vi "DemoVI_Thingworx.vi"() -> ()   [LabVIEW 2018]
panel:
  out "Thingworx Timestamp String":string="1557144000000"
  out "ThingworxTimestamp":dbl=1557144000000.0 format="%#_19g"
  out "Unix Timestamp":dbl=1557144000.0 format="%#_16g"
  in  "Labview Timestamp":timestamp=timestamp(3639960000 s since 1904-01-01) format="%<%H:%M:%S%3u\n%x>T"
  in  "Outer JSON":string
  in  "Inner JSON":string="StringField"
  in  "Outer JSON":string="rows"
  out "Complete Request URL":string="http://192.168.1.144:80/Thingworx/Things/LabviewTestObject/Properties/StringField"
  out "REST Answer as JSON 4":string="{\"dataShape\":{\"fieldDefinitions\":{\"result\":{\"name\":\"result\",\"description\":\"\",\"baseType\":\"STRING\",\"ordinal\":0,\"aspects\":{}}}},\"rows\":[{\"result\":\"input correct - service executed\"}]}"
  out "error out":errorcluster={"status"=FALSE, "code"=200, "source"="HTTP OK"}
  out "parsed JSON result --- jsonObject.row[0].result":string="input correct - service executed"
  in  "Thingworx Server Information":T1={"Server Adress"="192.168.1.144", "Port"="80", "http / https"="http", "Application Key"="8f240f9e-5025-45fe-9253-3b420d7beb56", "Entity Collection"="Things", "Name of Entity"="LabviewTestObject", "Characteristic Collection"="Services", "Name of Characteristic"="TestService", "Request Method"=enum."POST", "JSON Request Body"="{\n\"contentCheck\" : true\n}"}
  out "REST Answer as JSON 3":string="{\"dataShape\":{\"fieldDefinitions\":{\"result\":{\"name\":\"result\",\"description\":\"result\",\"baseType\":\"STRING\",\"ordinal\":0,\"aspects\":{}}}},\"rows\":[{\"result\":\"RUNNING\"}]}"
  out "error out":errorcluster={"status"=FALSE, "code"=200, "source"="HTTP OK"}
  out "parsed JSON result --- jsonObject.row[0].result":string="RUNNING"
  in  "Thingworx Server Information":T1={"Server Adress"="192.168.1.144", "Port"="80", "http / https"="http", "Application Key"="8f240f9e-5025-45fe-9253-3b420d7beb56", "Entity Collection"="Subsystems", "Name of Entity"="PlatformSubsystem", "Characteristic Collection"="Services", "Name of Characteristic"="GetSubsystemState", "Request Method"=enum."POST", "JSON Request Body"=""}
  out "REST Answer as JSON 2":string="{}"
  out "error out":errorcluster
  out "parsed JSON result --- not possible for put":string="***no result***"
  in  "Thingworx Server Information":T1={"Server Adress"="192.168.1.144", "Port"="80", "http / https"="http", "Application Key"="8f240f9e-5025-45fe-9253-3b420d7beb56", "Entity Collection"="Things", "Name of Entity"="LabviewTestObject", "Characteristic Collection"="Properties", "Name of Characteristic"="Timestamp", "Request Method"=enum."PUT", "JSON Request Body"="************This will be overwritten with the created Timestamp*********"}
  out "REST Answer as JSON":string="{\"dataShape\":{\"fieldDefinitions\":{\"StringField\":{\"name\":\"StringField\",\"description\":\"\",\"baseType\":\"STRING\",\"ordinal\":3,\"aspects\":{\"isPersistent\":true,\"dataChangeType\":\"VALUE\",\"cacheTime\":0.0}}}},\"rows\":[{\"StringField\":\"Custom String\"}]}"
  out "error out":errorcluster={"status"=FALSE, "code"=200, "source"="HTTP OK"}
  out "parsed JSON result --- jsonObject.rows[0].StringField":string="Custom String"
  in  "Thingworx Server Information":T1={"Server Adress"="192.168.1.144", "Port"="80", "http / https"="http", "Application Key"="8f240f9e-5025-45fe-9253-3b420d7beb56", "Entity Collection"="Things", "Name of Entity"="LabviewTestObject", "Characteristic Collection"="Properties", "Name of Characteristic"="StringField", "Request Method"=enum."GET", "JSON Request Body"=""}
  # "Demonstration of a GET call to retrieve propery values from Thingworx"
  # "Demonstration of a PUT call to set propery values in Thingworx"
  # "Demonstration of a POST call to execute a Thingworx service"
  # "Demonstration of a POST call to execute a Thingworx service with request body"
  # "If Outer JSON is empty, no JSON evaluation happens"
  # "The Thingworx Timestamp is the UNIX timestamp * 1000 to have the timestamp\nin milliseconds.\nThe epoch of Thingworx is 1/1/1970 in MS; the epoch of LabVIEW is 1/1/1904.\nTo help convert the dates, the SubVI Helper_Timestamp will do the transformation."
  # "Inner JSON and Outer JSON can be used to navigate \ndifferent than rows[0].result"
  # "Thingworx REST - Learning Guide"
  # "https://developer.thingworx.com/en/resources/guides/thingworx-rest-api-quickstart"
  # "Thingworx REST API Pattern"
  # "Thingworx REST API HTTP request verbs"
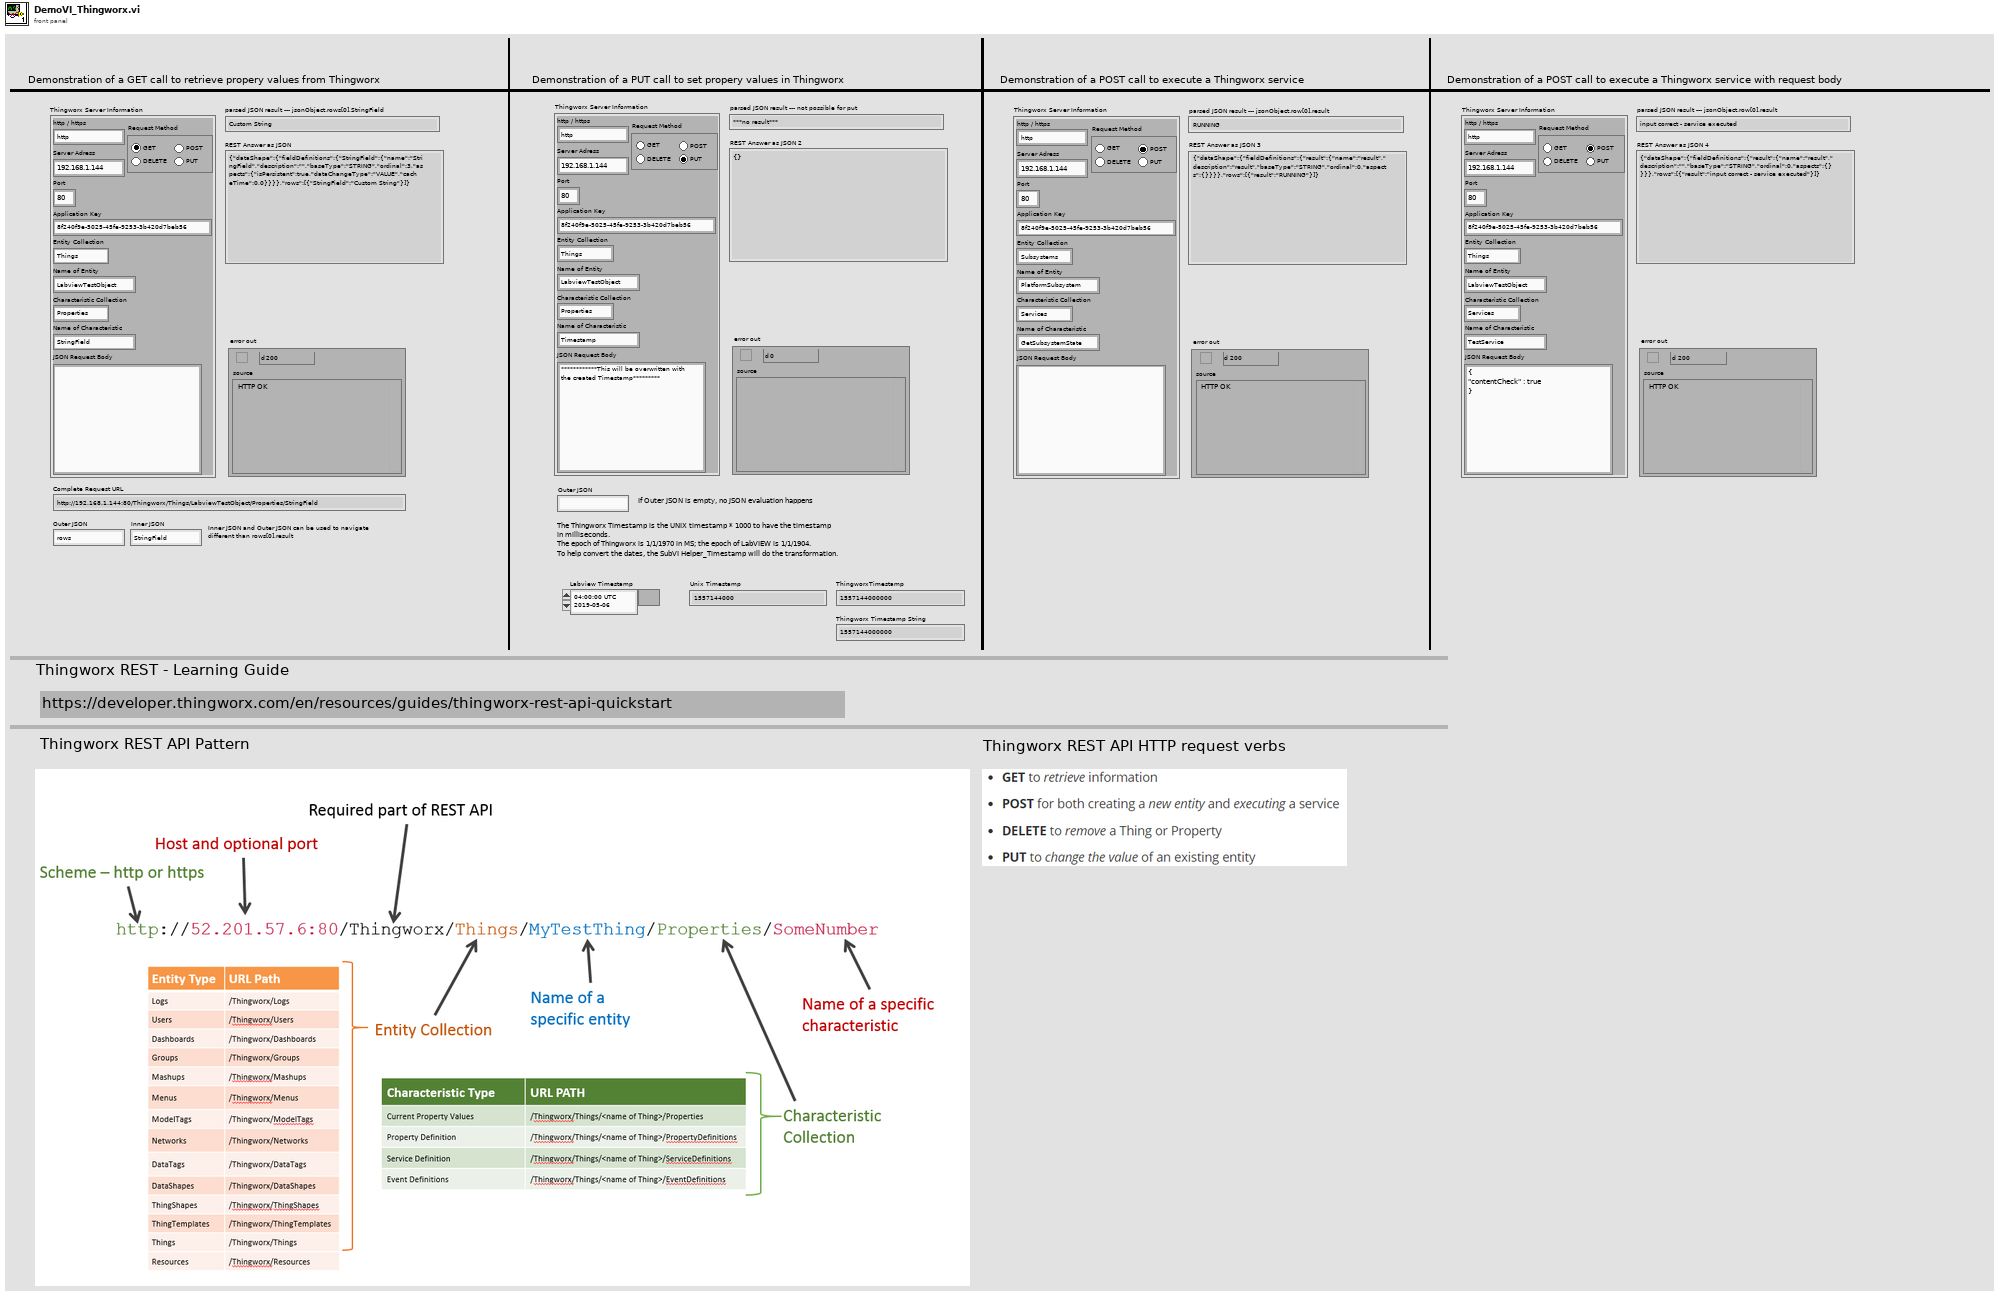
[diagram p1: front panel]
types:
  T1 = cluster{"Server Adress":string, "Port":string, "http / https":string, "Application Key":string, "Entity Collection":string, "Name of Entity":string, "Characteristic Collection":string, "Name of Characteristic":string, "Request Method":enum32{"GET", "POST", "DELETE", "PUT"}, "JSON Request Body":string}
  T2 = typedef "LabVIEWHTTPClient.lvlib/ClientHandle.ctl" = refnum<k1>
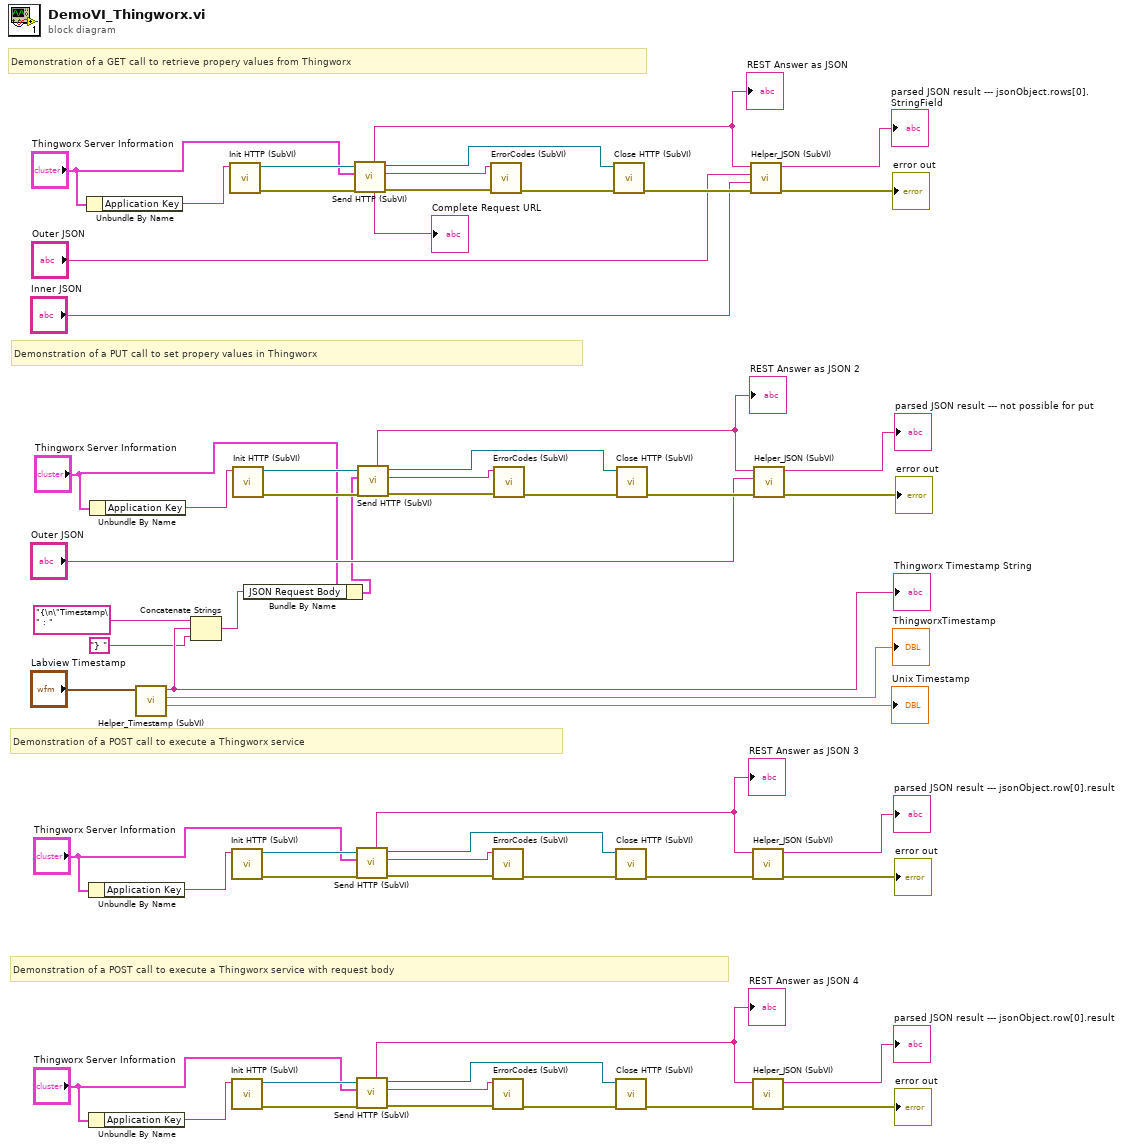
[diagram p0: block diagram]
diagram:
  # "Demonstration of a POST call to execute a Thingworx service with request body"
  # "Demonstration of a POST call to execute a Thingworx service"
  # "Demonstration of a PUT call to set propery values in Thingworx"
  # "Demonstration of a GET call to retrieve propery values from Thingworx"
  n1 = Unbundle By Name("Thingworx Server Information") -> ("Application Key"=w56:string)
  n2 = Unbundle By Name("Thingworx Server Information") -> ("Application Key"=w33:string)
  n3 = Unbundle By Name("Thingworx Server Information") -> ("Application Key"=w21:string)
  n4 = Unbundle By Name("Thingworx Server Information") -> ("Application Key"=w44:string)
  n5 = call "Helper_Timestamp (SubVI).vi"("Labview Timestamp"="Labview Timestamp") -> ("Unix Timestamp"=→"Unix Timestamp":dbl, "ThingworxTimestamp"=→"ThingworxTimestamp":dbl, "Thingworx Timestamp String"=w2:string)  [unwired: 8 in]
  "Thingworx Timestamp String" <- w2
  n6 = Concatenate Strings("{\n\"Timestamp\" : ", w2, "} ") -> (w4:string)
  n7 = call "Init HTTP (SubVI).vi"("Application Key"=w56) -> ("error out"=w54:errorcluster, "Refnum out"=w55:T2)  [unwired: 9 in]
  n8 = call "Init HTTP (SubVI).vi"("Application Key"=w33) -> ("error out"=w31:errorcluster, "Refnum out"=w32:T2)  [unwired: 9 in]
  n9 = call "Init HTTP (SubVI).vi"("Application Key"=w21) -> ("error out"=w19:errorcluster, "Refnum out"=w20:T2)  [unwired: 9 in]
  n10 = call "Init HTTP (SubVI).vi"("Application Key"=w44) -> ("error out"=w42:errorcluster, "Refnum out"=w43:T2)  [unwired: 9 in]
  n11 = Bundle By Name(cluster="Thingworx Server Information", "JSON Request Body"=w4) -> (w5:T1)
  n12 = call "Send HTTP (SubVI).vi"("error in (no error)"=w54, "Thingworx Server Information"="Thingworx Server Information", "Refnum in"=w55) -> ("error out"=w52:errorcluster, "headers"=w51:string, "Refnum out"=w50:T2, "Complete Request URL"=→"Complete Request URL":string, "body"=w49:string)  [unwired: 3 in, 1 out]
  "REST Answer as JSON" <- w49
  n13 = call "Send HTTP (SubVI).vi"("error in (no error)"=w31, "Thingworx Server Information"="Thingworx Server Information", "Refnum in"=w32) -> ("error out"=w29:errorcluster, "headers"=w28:string, "Refnum out"=w27:T2, "body"=w26:string)  [unwired: 3 in, 2 out]
  "REST Answer as JSON 3" <- w26
  n14 = call "Send HTTP (SubVI).vi"("error in (no error)"=w19, "Thingworx Server Information"="Thingworx Server Information", "Refnum in"=w20) -> ("error out"=w17:errorcluster, "headers"=w16:string, "Refnum out"=w15:T2, "body"=w14:string)  [unwired: 3 in, 2 out]
  "REST Answer as JSON 4" <- w14
  n15 = call "Send HTTP (SubVI).vi"("error in (no error)"=w42, "Thingworx Server Information"=w5, "Refnum in"=w43) -> ("error out"=w41:errorcluster, "headers"=w40:string, "Refnum out"=w39:T2, "body"=w38:string)  [unwired: 3 in, 2 out]
  "REST Answer as JSON 2" <- w38
  n16 = call "ErrorCodes (SubVI).vi"("error in (no error)"=w52, "Input"=w51) -> ("error out"=w58:errorcluster)  [unwired: 9 in]
  n17 = call "ErrorCodes (SubVI).vi"("error in (no error)"=w29, "Input"=w28) -> ("error out"=w35:errorcluster)  [unwired: 9 in]
  n18 = call "ErrorCodes (SubVI).vi"("error in (no error)"=w17, "Input"=w16) -> ("error out"=w23:errorcluster)  [unwired: 9 in]
  n19 = call "ErrorCodes (SubVI).vi"("error in (no error)"=w41, "Input"=w40) -> ("error out"=w46:errorcluster)  [unwired: 9 in]
  n20 = call "Close HTTP (SubVI).vi"("error in (no error)"=w58, "Refnum in"=w50) -> ("error out"=w59:errorcluster)  [unwired: 9 in]
  n21 = call "Close HTTP (SubVI).vi"("error in (no error)"=w35, "Refnum in"=w27) -> ("error out"=w36:errorcluster)  [unwired: 9 in]
  n22 = call "Close HTTP (SubVI).vi"("error in (no error)"=w23, "Refnum in"=w15) -> ("error out"=w24:errorcluster)  [unwired: 9 in]
  n23 = call "Close HTTP (SubVI).vi"("error in (no error)"=w46, "Refnum in"=w39) -> ("error out"=w47:errorcluster)  [unwired: 9 in]
  n24 = call "Helper_JSON (SubVI).vi"("error in (no error)"=w59, "Inner JSON"="Inner JSON", "Outer JSON"="Outer JSON", "body"=w49) -> ("error out"=→"error out":errorcluster, "String Value"=→"parsed JSON result --- jsonObject.rows[0].StringField":string)  [unwired: 6 in]
  n25 = call "Helper_JSON (SubVI).vi"("error in (no error)"=w36, "body"=w26) -> ("error out"=→"error out":errorcluster, "String Value"=→"parsed JSON result --- jsonObject.row[0].result":string)  [unwired: 8 in]
  n26 = call "Helper_JSON (SubVI).vi"("error in (no error)"=w24, "body"=w14) -> ("error out"=→"error out":errorcluster, "String Value"=→"parsed JSON result --- jsonObject.row[0].result":string)  [unwired: 8 in]
  n27 = call "Helper_JSON (SubVI).vi"("error in (no error)"=w47, "Outer JSON"="Outer JSON", "body"=w38) -> ("error out"=→"error out":errorcluster, "String Value"=→"parsed JSON result --- not possible for put":string)  [unwired: 7 in]
